vi "Ref Signal.vi"(1 "Samples [n]":i32) -> (4 "Ref [n]":dbl, 5 "RefDot [n]":dbl format="%0.2f")   [LabVIEW 2013]
uses:
  <vilib>/ptbypt/NI_PtbyPt.lvlib
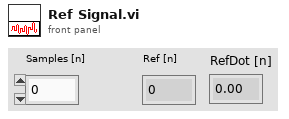
[diagram p1: front panel]
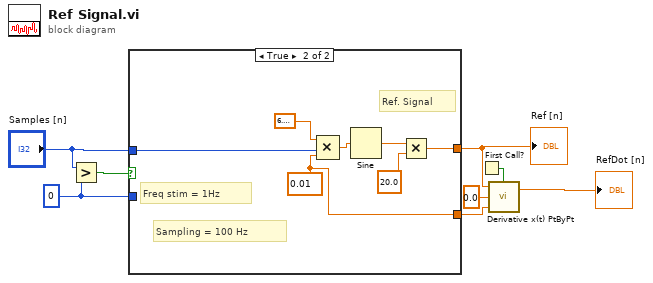
[diagram p0: block diagram]
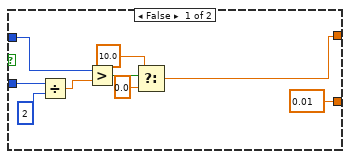
[diagram p2: hidden frame]
diagram:
  w1 = 0 ("y")
  n1 = Greater?(x="Samples [n]", y=w1) -> (0:w2:bool)
  n2 = case shown="True" w2 {
    tunnel: "Samples [n]" -> [w16 w20]
    tunnel: [w9 w19] -> w8
    tunnel: [0.01 ("y") w18] -> w5
    tunnel: w1 -> [w15 _]
    frame False {
      n3 = Divide(x=w15, y=2) -> (x/y=w14:dbl)
      n4 = Greater?(x=w16, y=w14) -> (0:w12:bool)
      n5 = Select(t=10.0, s=w12, f=0.0) -> (s? t:f=w9:dbl)
    }
    frame True {
      w18 = 0.01 ("y")
      # "Freq stim = 1Hz"
      # "Sampling = 100 Hz"
      # "Ref. Signal"
      n6 = Compound Arithmetic op=MULTIPLY(6.283185307179586, w20, w18) -> (w21:dbl)
      n7 = Sine(x=w21) -> (sin(x)=w23:dbl)
      n8 = Multiply(x=w23, y=20.0) -> (x*y=w19:dbl)
    }
  }
  "Ref [n]" <- w8
  n9 = First Call?() -> (First Call?: T/F=w7:bool)
  n10 = call <vilib>:"Derivative x(t) PtByPt.vi"("initialize"=w7, "dt"=w5, "initial condition"=0.0, "x"=w8) -> ("dx/dt"=→"RefDot [n]":dbl)  [unwired: 1 out]
